vi "Resolve Moves.vi"(6 "Teams in":refnum<class "Team.lvclass">[](array[class]), 9 "New Map in":refnum<class "Map.lvclass">, 11 "Map in":refnum<class "Map.lvclass">) -> (1 "New Map out":refnum<class "Map.lvclass">, 4 "Teams out":refnum<class "Team.lvclass">[](array[class]))   [LabVIEW 2020, in "SquareBattle.lvlib" / "Map.lvclass"]
uses:
  Map.lvclass
  Team/Team.lvclass
  Map.lvclass/Map.ctl
  Position.ctl
  Action.ctl
  Square/Square.lvclass
  Direction Position Offsets.vi
  Normalize Position.vi
  SquareBattle.lvlib
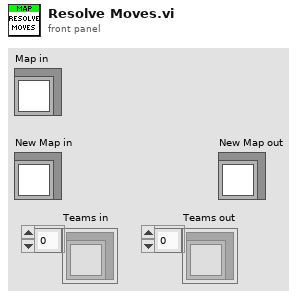
[diagram p1: front panel]
types:
  T1 = typedef "SquareBattle.lvlib/Position.ctl" = cluster{"Row":i32, "Col":i32}
  T2 = typedef "SquareBattle.lvlib/Action.ctl" = enum16{"Wait", "Move", "Attack", "Replicate"}
  T3 = typedef "SquareBattle.lvlib/Run Result.ctl" = cluster{"Action":T2, "Direction":T4, "Replication":refnum<class "Square.lvclass">}
  T4 = typedef "SquareBattle.lvlib/Direction.ctl" = enum16{"NW", "N", "NE", "E", "SE", "S", "SW", "W"}
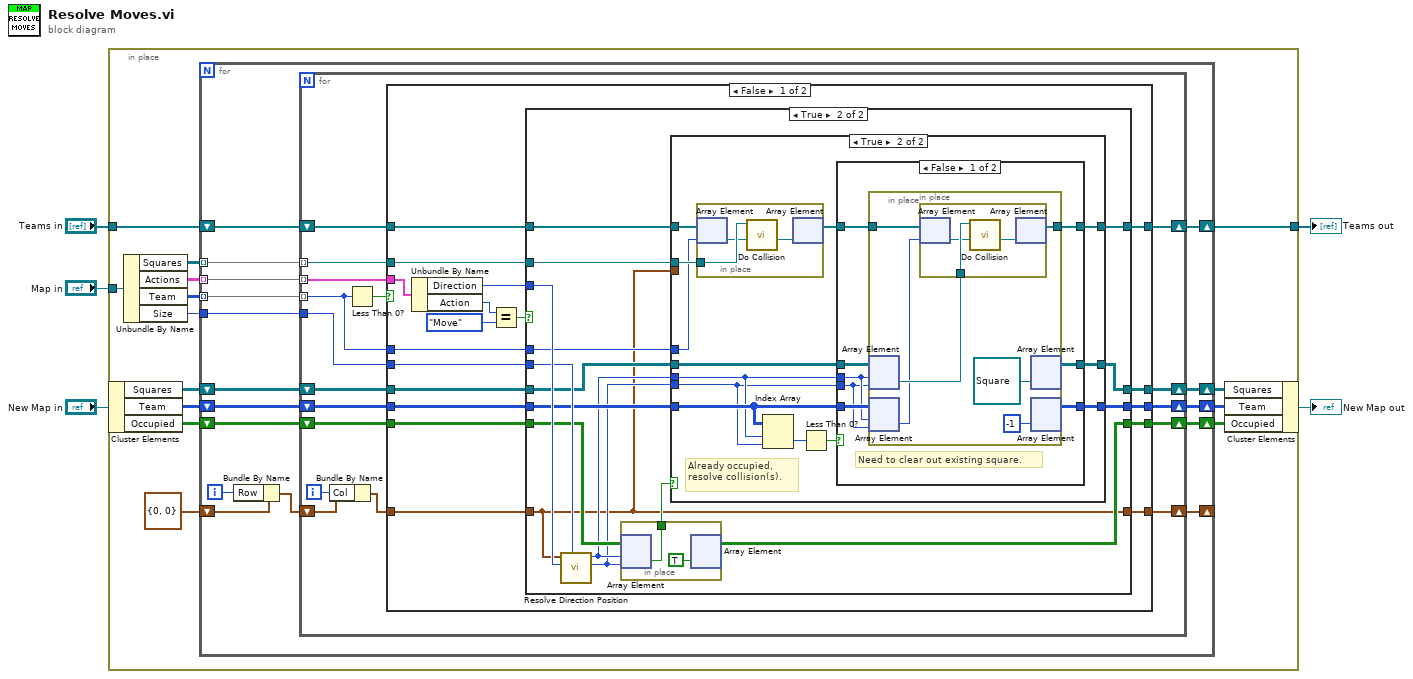
[diagram p0: block diagram]
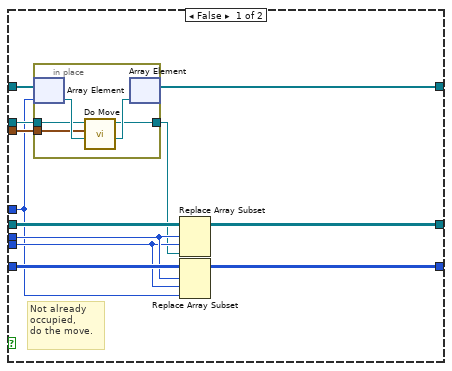
[diagram p3: hidden frame]
diagram:
  n1 = in-place {
    in-place-border: "Map in" -> [w19]
    in-place-border: "Teams in" -> [w7]
    in-place-border: [w6] -> w1
    n2 = in-place-cluster #1("New Map in") -> ("Squares"=w15:refnum<class "Square.lvclass">[][], "Team"=w14:i32[][], "Occupied"=w13:bool[][])
    n3 = Unbundle By Name(w19) -> ("Squares"=w18:refnum<class "Square.lvclass">[][], "Actions"=w17:T3[][], "Team"=w16:i32[][], "Size"=w8:i32)
    n4 = for {
      tunnel: w18 -> [w35] mode=indexing
      tunnel: w17 -> [w34] mode=indexing
      tunnel: w16 -> [w33] mode=indexing
      shift-right: [w27] -> w12
      shift-left: w15 -> [w32]
      shift-right: [w29] -> w11
      shift-left: w13 -> [w30]
      shift-right: [w28] -> w10
      shift-left: w14 -> [w31]
      tunnel: w8 -> [w25]
      shift-right: [w22] -> _
      shift-left: T1 {"Row"=0, "Col"=0} ("Position") -> [w24]
      shift-right: [w20] -> w6
      shift-left: w7 -> [w21]
      i -> [w26]
      n5 = Bundle By Name(cluster=w24, "Row"=w26) -> (w23:T1)
      n6 = for {
        tunnel: w35 -> [w49] mode=indexing
        tunnel: w34 -> [w50] mode=indexing
        tunnel: w33 -> [w51] mode=indexing
        shift-right: [w48] -> w27
        shift-left: w32 -> [w47]
        shift-right: [w44] -> w29
        shift-left: w30 -> [w43]
        shift-right: [w46] -> w28
        shift-left: w31 -> [w45]
        tunnel: w25 -> [w39]
        shift-right: [w38] -> w22
        shift-left: w23 -> [w42]
        shift-right: [w36] -> w20
        shift-left: w21 -> [w37]
        i -> [w41]
        n7 = Bundle By Name(cluster=w42, "Col"=w41) -> (w40:T1)
        n8 = Less Than 0?(x=w51) -> (x < 0?=w52:bool)
        n9 = case shown="False" w52 {
          tunnel: w51 -> [w58 _]
          tunnel: w50 -> [w70 _]
          tunnel: w49 -> [w67 _]
          tunnel: [w64 w151] -> w48
          tunnel: w47 -> [w63 w151]
          tunnel: [w62 w150] -> w46
          tunnel: w45 -> [w61 w150]
          tunnel: [w60 w149] -> w44
          tunnel: w43 -> [w59 w149]
          tunnel: w40 -> [w57 w148]
          tunnel: w39 -> [w56 _]
          tunnel: [w55 w148] -> w38
          tunnel: w37 -> [w54 w147]
          tunnel: [w53 w147] -> w36
          frame False {
            n10 = Unbundle By Name(w70) -> ("Direction"=w66:T4, "Action"=w69:T2)
            n11 = Equal?(x=w69, y=Action."Move") -> (x = y?=w65:bool)
            n12 = case shown="True" w65 {
              tunnel: w67 -> [_ w84]
              tunnel: w66 -> [_ w91]
              tunnel: [w75 w81] -> w64
              tunnel: w63 -> [w75 w86]
              tunnel: [w74 w82] -> w62
              tunnel: w61 -> [w74 w87]
              tunnel: [w73 w88] -> w60
              tunnel: w59 -> [w73 w89]
              tunnel: w58 -> [_ w83]
              tunnel: w57 -> [w72 w76]
              tunnel: w56 -> [_ w90]
              tunnel: [w72 w76] -> w55
              tunnel: w54 -> [w71 w78]
              tunnel: [w71 w77] -> w53
              frame False {
                # "Not a move, do nothing."
              }
              frame True {
                n13 = call "Resolve Direction Position.vi"("Board Size"=w90, "Direction"=w91, "From"=w76) -> ("Col"=w79:i32, "Row"=w80:i32)  [unwired: 6 in, 1 out]
                n14 = in-place {
                  in-place-border: [w146] -> w85
                  n15 = in-place-array #2(w89, w80, w79) -> (w146:bool)
                  n16 = in-place-array #2(TRUE ("element")) -> (w88:bool[][])  [unwired: 2 out]
                }
                n17 = case shown="True" w85 {
                  tunnel: w87 -> [w103 w115]
                  tunnel: w86 -> [w101 w118]
                  tunnel: w84 -> [w96 w121]
                  tunnel: w83 -> [w92 w113]
                  tunnel: [w102 w116] -> w82
                  tunnel: [w100 w117] -> w81
                  tunnel: w80 -> [w99 w112]
                  tunnel: w79 -> [w98 w111]
                  tunnel: w78 -> [w97 w114]
                  tunnel: [w94 w109] -> w77
                  tunnel: w76 -> [w95 _]
                  frame False {
                    # "Not already occupied,\ndo the move."
                    n18 = in-place {
                      in-place-border: w96 -> [w107]
                      in-place-border: w95 -> [w106]
                      in-place-border: [w104] -> w93
                      n19 = in-place-array #3(w97, w92) -> (w108:refnum<class "Team.lvclass">)
                      n20 = call "Do Move.vi"("Team in"=w108, "Position"=w106, "Square in"=w107) -> ("Team out"=w105:refnum<class "Team.lvclass">, "Square out"=w104:refnum<class "Square.lvclass">)  [unwired: 7 in]
                      n21 = in-place-array #3(w105) -> (w94:refnum<class "Team.lvclass">[])  [unwired: 1 out]
                    }
                    n22 = Replace Array Subset(array=w101, new element=w93, index (row)=w99, index (col)=w98) -> (w100:refnum<class "Square.lvclass">[][])
                    n23 = Replace Array Subset(array=w103, new element=w92, index (row)=w99, index (col)=w98) -> (w102:i32[][])
                  }
                  frame True {
                    # "Already occupied, resolve collision(s)."
                    n24 = in-place {
                      in-place-border: w121 -> [w124]
                      n25 = in-place-array #4(w114, w113) -> (w123:refnum<class "Team.lvclass">)
                      n26 = call "Do Collision.vi"("Team in"=w123, "Square"=w124) -> ("Team out"=w122:refnum<class "Team.lvclass">)  [unwired: 9 in]
                      n27 = in-place-array #4(w122) -> (w110:refnum<class "Team.lvclass">[])  [unwired: 1 out]
                    }
                    n28 = Index Array(array=w115, index (row)=w112, index (col)=w111) -> (element=w120:i32)
                    n29 = Less Than 0?(x=w120) -> (x < 0?=w119:bool)
                    n30 = case shown="False" w119 {
                      tunnel: w118 -> [w132 w144]
                      tunnel: [w130 w144] -> w117
                      tunnel: [w125 w143] -> w116
                      tunnel: w115 -> [w129 w143]
                      tunnel: w112 -> [w128 _]
                      tunnel: w111 -> [w127 _]
                      tunnel: w110 -> [w131 w142]
                      tunnel: [w126 w142] -> w109
                      frame False {
                        # "Need to clear out existing square."
                        n31 = in-place {
                          in-place-border: w131 -> [w135]
                          in-place-border: [w134] -> w126
                          n32 = in-place-array #5(w132, w128, w127) -> (w136:refnum<class "Square.lvclass">)
                          n33 = in-place-array #6(w129, w128, w127) -> (w133:i32)
                          n34 = in-place {
                            in-place-border: w136 -> [w141]
                            n35 = in-place-array #7(w135, w133) -> (w140:refnum<class "Team.lvclass">)
                            n36 = call "Do Collision.vi"("Team in"=w140, "Square"=w141) -> ("Team out"=w139:refnum<class "Team.lvclass">)  [unwired: 9 in]
                            n37 = in-place-array #7(w139) -> (w134:refnum<class "Team.lvclass">[])  [unwired: 1 out]
                          }
                          n38 = in-place-array #5(refnum<class "Square.lvclass"> refnum ("element")) -> (w130:refnum<class "Square.lvclass">[][])  [unwired: 2 out]
                          n39 = in-place-array #6(-1 ("element")) -> (w125:i32[][])  [unwired: 2 out]
                        }
                      }
                      frame True {
                        # "Already emptied, don't need to handle collision for target."
                      }
                    }
                  }
                }
              }
            }
          }
          frame True {
            # "Empty, do nothing."
          }
        }
      }
    }
    n40 = in-place-cluster #1("Squares"=w12, "Team"=w10, "Occupied"=w11) -> (→"New Map out":refnum<class "Map.lvclass">)
  }
  "Teams out" <- w1
